vi "sub-Language-get str-const.vi"(1 "sid":u32 format="%04x") -> (0 "str":string)   [LabVIEW 2011]
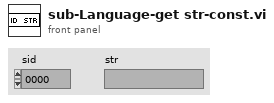
[diagram p1: front panel]
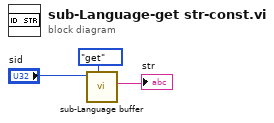
[diagram p0: block diagram]
diagram:
  n1 = call "sub-Language buffer.vi"("operation"=enum16{"clear", "add", "get"}."get", "ID"="sid") -> ("str out"=→"str":string)  [unwired: 8 in, 1 out]
